vi "NETCallback FileWatcher Broadcast.vi"(4 "User Parameter":T1, 5 "Event Data":cluster{"sender":refnum<k39>, "e":refnum<k39>}, 6 "Control Ref":refnum<k39>, 7 "Event Common Data":T2) -> ()   [LabVIEW 2026]
uses:
  C:/Program Files/dotnet/shared/Microsoft.NETCore.App/8.0.25/System.IO.FileSystem.Watcher.dll
  Program Files/dotnet/shared/Microsoft.NETCore.App/8.0.25/System.IO.FileSystem.Watcher.dll
  C:/Program Files/dotnet/shared/Microsoft.NETCore.App/8.0.25/System.Private.CoreLib.dll
  Program Files/dotnet/shared/Microsoft.NETCore.App/8.0.25/System.Private.CoreLib.dll
  5b99c23a-5df9-4087-89f4-512f78e848ed.vi
  <vilib>/JDP Science/JSONtext/Variant to JSON Text.vi
  <vilib>/JDP Science/JSONtext/LVClass Serializer/JSONtext LVClass Serializer.lvclass
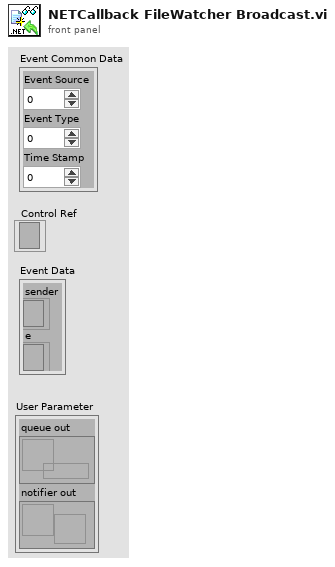
[diagram p1: front panel]
types:
  T1 = cluster{"queue out":refnum<queue>, "notifier out":refnum<notifier>}
  T2 = cluster{"Event Source":i32, "Event Type":u32, "Time Stamp":u32}
  T3 = cluster{"ToString":string, "ChangeType":i32, "FullPath":string, "Name":string}
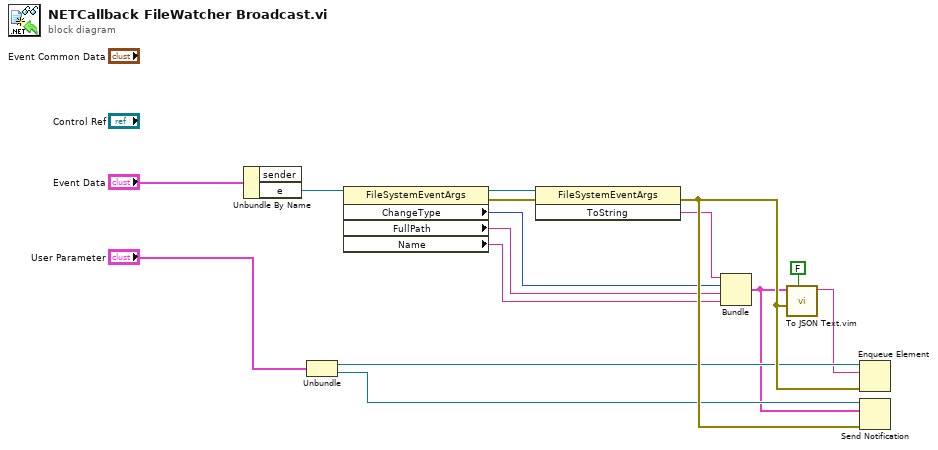
[diagram p0: block diagram]
diagram:
  n1 = Unbundle By Name("Event Data") -> ("e"=w13:refnum<k39>)  [unwired: 1 out]
  n2 = Unbundle("User Parameter") -> ("queue out"=w6:refnum<queue>, "notifier out"=w5:refnum<notifier>)
  n3 = property class="FileSystemEventArgs"(reference=w13) -> (reference out=w12:refnum<k39>, error out=w2:errorcluster, "ChangeType"=w10:i32, "FullPath"=w9:string, "Name"=w8:string)  [unwired: 1 in]
  n4 = invoke class="FileSystemEventArgs" method="ToString"(reference=w12, error in=w2) -> (error out=w15:errorcluster, "ToString"=w11:string)  [unwired: 1 in, 1 out]
  n5 = Bundle("ToString"=w11, "ChangeType"=w10, "FullPath"=w9, "Name"=w8) -> (w4:T3)  [unwired: 1 in]
  n6 = call "To JSON Text.vim"("enable LabVIEW extensions? (T)"=FALSE, "error in (no error)"=w15, "Anything"=w4) -> ("<JSON>"=w3:string)  [unwired: 7 in, 1 out]
  n7 = Enqueue Element(queue=w6, element=w3, error in (no error)=w15) -> ()  [unwired: 1 in, 3 out]
  n8 = Send Notification(notification=w4, notifier=w5, error in (no error)=w15) -> ()  [unwired: 2 out]
